vi "RT.vi"() -> ()   [LabVIEW 2017]
uses:
  <vilib>/Platform/TimedLoop/XDataNode/timing_clust.ctl
  <vilib>/Platform/TimedLoop/XDataNode/nitl_modes.ctl
  <vilib>/Platform/TimedLoop/XDataNode/wakeup.ctl
  <vilib>/FPGAPlugInAG/PXI-7852R/niLvFpga_Open_PXI-7852R.vi
  <vilib>/rvi/interface/common/dynamic/niFpgaDynamicAddResources.vi
  <vilib>/FPGAPlugInAG/Dynamic/niLvFpga_Run_Dynamic.vi
  <vilib>/Utility/error.llb/Error Cluster From Error Code.vi
  <vilib>/rvi/errors/niLvFpgaAdjustHostInterfaceError.vi
  <vilib>/FPGAPlugInAG/Dynamic/niLvFpga_Close_Dynamic.vi
  <vilib>/platform/TimedLoop/XDataNode/XDataNode.xnode
  <vilib>/rvi/interface/nirviOpenFPGA/nirviOpenFPGA.xnode
  FPGA Bitfiles/PXI_FPGATarget_FPGA_z50FCp+1-Jo.lvbitx
  FPGA.vi
  <vilib>/rvi/interface/nirviMethod/nirviMethod.xnode
  <vilib>/rvi/interface/nirviCloseFPGA/nirviCloseFPGA.xnode
  <vilib>/Platform/TimedLoop/XDataNode/XDNodeRunTimeDep.lvlib
  <vilib>/FPGAPlugInAG/Dynamic/niLvFpga_ReadFifo_Dynamic.vi
  <vilib>/rvi/errors/niLvFpgaMergeErrorWithErrorCode.vi
panel:
  in  "Stop FPGA?":bool
  in  "Period ms":i64=1000
  out "error out":errorcluster
  out "Elements Remaining":u32
  out "Data":sgl[](array[numeric])
  in  "stop":bool
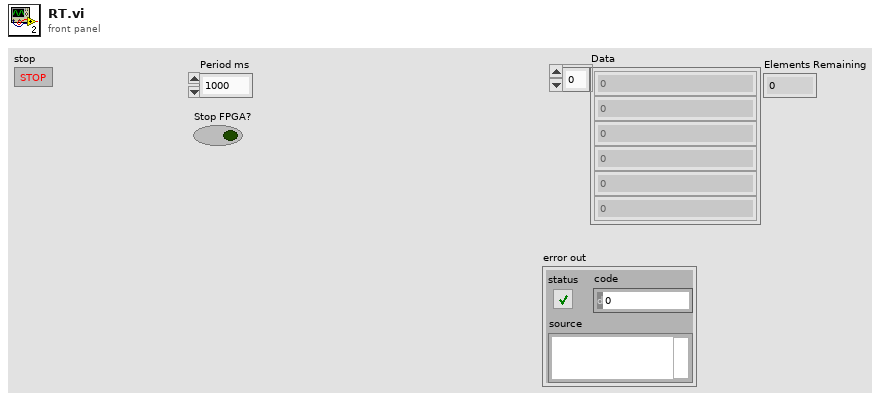
[diagram p1: front panel]
types:
  T1 = typedef "XDNodeRunTimeDep.lvlib/timing_clust.ctl" = cluster{"Expected End [f-1]":u64, "Actual End [f-1]":u64, "Finished Late? [f-1]":bool, "Expected End [i-1]":u64, "Actual End [i-1]":u64, "Finished Late? [i-1]":bool, "Expected Start [i]":u64, "Actual Start [i]":u64, "Expected Start [f]":u64, "Actual Start [f]":u64, "Source Name":string, "Structure Name":string, "Period":i64, "Deadline":i64, "Offset":i64, "Start":i64, "Priority":i32, "Timeout":i32, "Mode":T2, "Wakeup Reason":T3, "Error":errorcluster, "Source Type":string, "Secondary Source Type":string, "Global End Time":u64, "Global Start Time":u64, "Frame Duration":u64, "Iteration Duration":u64, "Assigned CPU":i32, "I/O Scan Engine Mode":u32}
  T2 = typedef "XDNodeRunTimeDep.lvlib/nitl_modes.ctl" = enum32{"No Change", "Process missed periods, maintain original phase", "Discard missed periods, maintain original phase", "Process missed periods, ignore original phase", "Discard missed periods, ignore original phase"}
  T3 = typedef "XDNodeRunTimeDep.lvlib/wakeup.ctl" = enum32{"Normal", "Aborted", "Asynchronous wakeup", "Timing source error", "Timed loop error", "Timeout"}
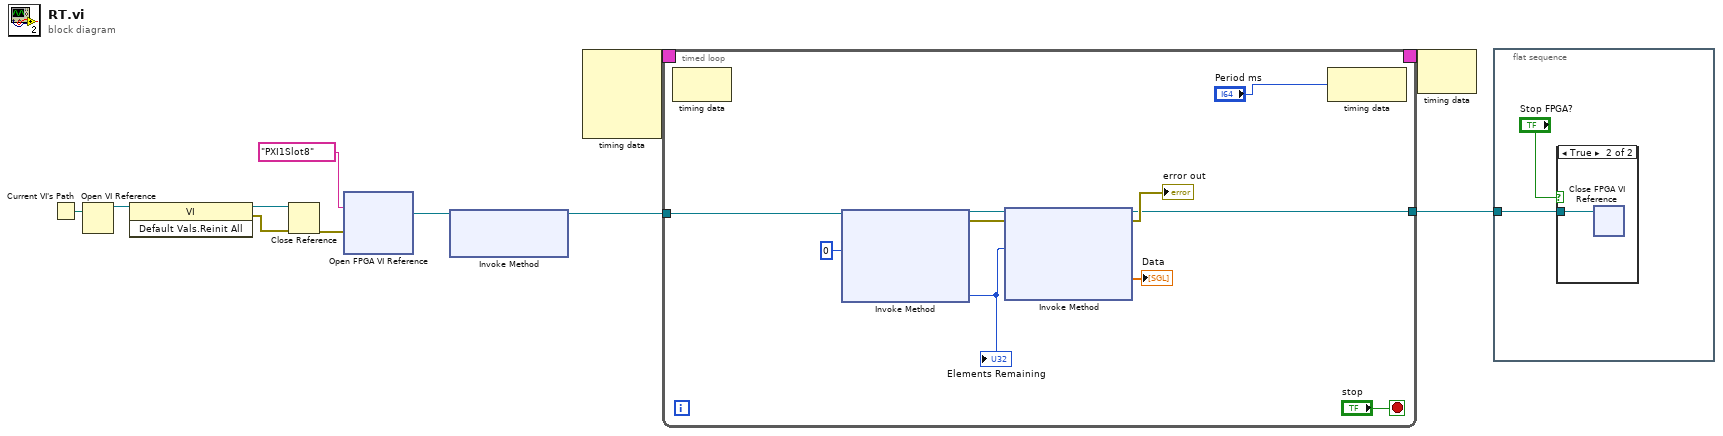
[diagram p0: block diagram]
diagram:
  n1 = Current VI's Path() -> (path=w5:path)
  n2 = Open VI Reference(vi path=w5) -> (vi reference=w6:refnum<vi>)  [unwired: 5 in, 1 out]
  n3 = invoke class="VI" method="Default Vals.Reinit All"(reference=w6) -> (reference out=w4:refnum<vi>, error out=w3:errorcluster)  [unwired: 2 in, 1 out]
  n4 = Close Reference(reference=w4, error in (no error)=w3) -> (error out=w2:errorcluster)
  n5 = xnode "Open FPGA VI Reference"("error in"=w2, "resource name"=tag "PXI1Slot8") -> ("FPGA VI Reference Out"=w9:refnum<k20>)  [unwired: 1 out]
  n6 = xnode "Invoke Method"("FPGA VI Reference In"=w9) -> ("FPGA VI Reference Out"=w8:refnum<k20>)  [unwired: 2 in, 1 out]
  n7 = node-c288() -> (w11:T1)  [unwired: 4 in]
  n8 = timed-loop {
    timing: w11 -> [_]
    timing-out: [_] -> w10
    tunnel: w8 -> [w21]
    tunnel: [w13] -> w7
    stop <- "stop" stop-if-true
    n9 = node-c288() -> ()  [unwired: 1 in, 1 out]
    n10 = xnode "Invoke Method"("FPGA VI Reference In"=w21, "Number of Elements"=u32 0) -> ("FPGA VI Reference Out"=w18:refnum<k20>, "error out"=w15:errorcluster, "Elements Remaining"=w19:u32)  [unwired: 2 in, 1 out]
    "Elements Remaining" <- w19
    n11 = xnode "Invoke Method"("FPGA VI Reference In"=w18, "error in"=w15, "Number of Elements"=w19) -> ("FPGA VI Reference Out"=w13:refnum<k20>, "error out"=→"error out":errorcluster, "Data"=→"Data":sgl[])  [unwired: 1 in, 1 out]
    n12 = node-c288("Period ms") -> ()  [unwired: 1 out]
  }
  n13 = node-c288(w10) -> ()  [unwired: 1 out]
  n14 = flat-sequence {
    tunnel: w7 -> [w27]
    frame #0 {
      n15 = case shown="True" "Stop FPGA?" {
        tunnel: w27 -> [_ w28]
        frame False {
        }
        frame True {
          n16 = xnode "Close FPGA VI Reference"("FPGA VI Reference In"=w28) -> ()  [unwired: 1 in, 1 out]
        }
      }
    }
  }
